vi "TLPM Initialize.vi"(8 "error in (no error)":errorcluster {"code" format="%.0x"}, 9 "Reset Device (Reset Device)":bool=TRUE, 10 "ID Query (Do Query)":bool=TRUE, 11 "resource name":refnum<visa-resource-name>) -> (0 "error out":errorcluster {"code" format="%.0x"}, 3 "instrument handle out":refnum<visa-resource-name>)   [LabVIEW 2019]
doc: "This VI initializes the instrument driver session and performs the following initialization actions:\n\n(1) Opens a session to the Default Resource Manager resource and a session to the specified device using the Resource Name.\n(2) Performs an identification query on the instrument.\n(3) Resets the instrument to a known state.\n(4) Sends initialization commands to the instrument.\n(5) Returns an instrument handle which is used to distinguish between different sessions of this instrument driver.\n\nNotes:\n(1) Each time this VI is invoked a unique session is opened."
uses:
  TLPM_32.dll
panel:
  # "(C) 2021 National Instruments.  ALL RIGHTS RESERVED."
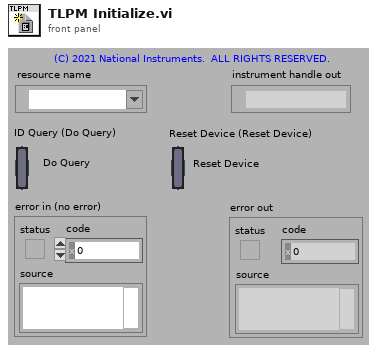
[diagram p1: front panel]
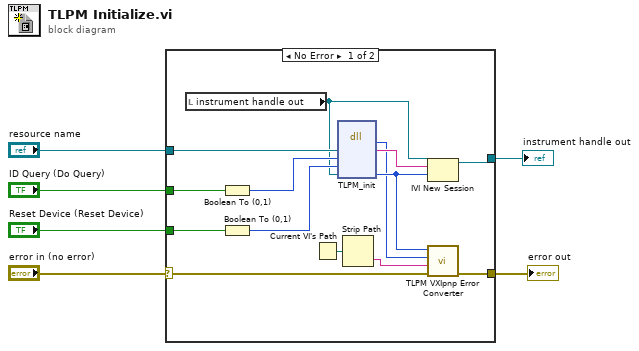
[diagram p0: block diagram]
diagram:
  n1 = case shown="No Error" "error in (no error)" {
    selector: "error in (no error)" -> [w8 w21]
    tunnel: [w7 w21] -> w5
    tunnel: "resource name" -> [w16 _]
    tunnel: [w15 _] -> w3
    tunnel: "ID Query (Do Query)" -> [w13 _]
    tunnel: "Reset Device (Reset Device)" -> [w12 _]
    frame No Error {
      n2 = local read "instrument handle out"() -> (w14:refnum<visa-resource-name>)
      n3 = Boolean To (0,1)(Boolean=w13) -> (0, 1=w20:i16)
      n4 = Boolean To (0,1)(Boolean=w12) -> (0, 1=w19:i16)
      n5 = Current VI's Path() -> (path=w17:path)
      n6 = dll-call lib="TLPM_32.dll" fn="TLPM_init"("resource name"=w16, "id query"=w20, "reset device"=w19, "instrument handle"=w14) -> ("status"=w10:i32, "resource name"=w18:string, "instrument handle"=w11:u32)  [unwired: 5 in, 2 out]
      n7 = Strip Path(path=w17) -> (name=w9:string)  [unwired: 1 out]
      n8 = IVI New Session(9:w11, 10:w18, 11:w14) -> (3:w15:refnum<visa-resource-name>)
      n9 = call <userlib>:"TLPM VXIpnp Error Converter.vi"("error in (no error)"=w8, "Name Of VI (\"\")"=w9, "CVI Error Code (0)"=w10, "instrument handle"=w11) -> ("error out"=w7:errorcluster)  [unwired: 6 in, 1 out]
    }
    frame Error {
    }
  }
  "error out" <- w5
  "instrument handle out" <- w3
